vi "login test.vi"   [LabVIEW 2014]
uses:
  <vilib>/httpClient/LabVIEWHTTPClient.lvlib
  <vilib>/httpClient/POSTBuffer.vi
types:
  T1 = typedef "LabVIEWHTTPClient.lvlib/ClientHandle.ctl" = refnum<k1>
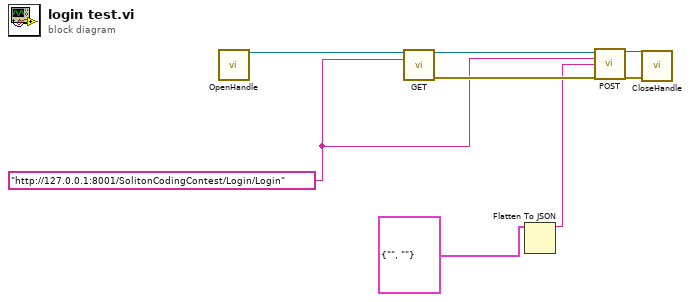
[diagram p0: block diagram]
diagram:
  w3 = "http://127.0.0.1:8001/SolitonCodingContest/Login/Login" ("url")
  n1 = call <vilib>:"OpenHandle.vi"() -> ("client handle out"=w7:T1)  [unwired: 14 in, 1 out]
  n2 = call <vilib>:"GET.vi"("client handle"=w7, "url"=w3) -> ("client handle out"=w5:T1, "error out"=w6:errorcluster)  [unwired: 10 in, 2 out]
  n3 = Flatten To JSON(anything=cluster{"userName":string, "password":string} {"userName"="", "password"=""}) -> (JSON string=w1:string)  [unwired: 2 in, 1 out]
  n4 = call-poly <vilib>:"POST.vi"("client handle"=w5, "url"=w3, "buffer"=w1) -> ("client handle out"=w4:T1)  [unwired: 9 in, 3 out]
  n5 = call <vilib>:"CloseHandle.vi"("client handle"=w4, "error in (no error)"=w6) -> ()  [unwired: 13 in, 1 out]
